vi "Write File Name.vi"(8 "error in (no error)":errorcluster, 10 "File Name":string, 11 "EMG in":refnum<class "EMG.lvclass">) -> (0 "error out":errorcluster, 3 "EMG out":refnum<class "EMG.lvclass">)   [LabVIEW 2014]
uses:
  EMG.lvclass
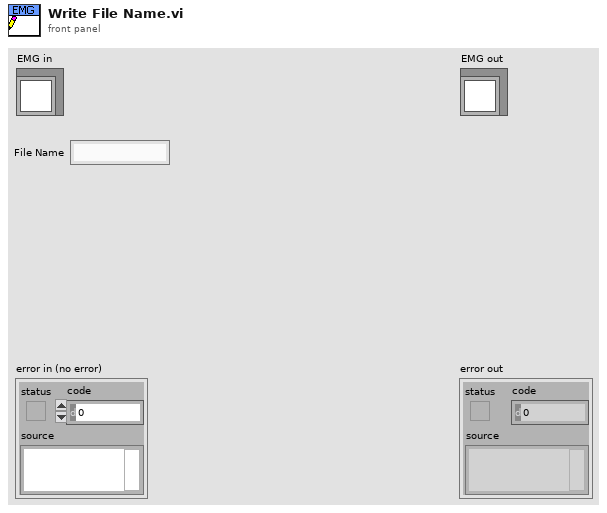
[diagram p1: front panel]
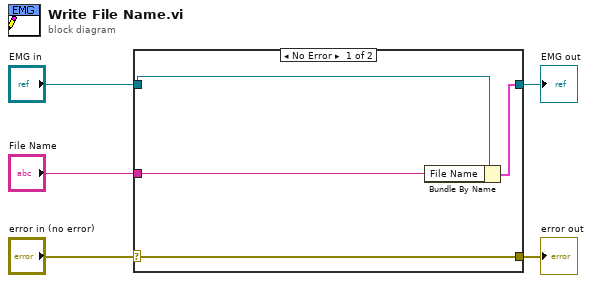
[diagram p0: block diagram]
diagram:
  n1 = case shown="No Error" "error in (no error)" {
    selector: "error in (no error)" -> [w9 w10]
    tunnel: [w9 w10] -> w4
    tunnel: [w7 w11] -> w2
    tunnel: "EMG in" -> [w8 w11]
    tunnel: "File Name" -> [w6 _]
    frame No Error {
      n2 = Bundle By Name(cluster=w8, "File Name"=w6) -> (w7:cluster{})
    }
    frame Error {
    }
  }
  "error out" <- w4
  "EMG out" <- w2
